vi "Process BMP JPG PNG.vi"() -> ()   [LabVIEW 2015]
uses:
  Typedefs/typedef_enum_ColorSpace.ctl
  Typedefs/typedef_enum_RGB HSL.ctl
panel:
  in  "Threshhold":i32=100
  out "Image_Object":i16[][](graph)
  out "Object(s) Start/Stop/Sum":i32[][](array[numeric])
  in  "cumulative?":bool
  out "RGB/HSL":T1[](array[typedef])=[enum."Red/Hue", enum."Grn/Sat", enum."Blu/Lit"]
  out "Col_Sum":cluster{i32[], "Col_Sum":i16[]}(graph)
  out "Row_Sum":cluster{"Row_Sum":i16[], i32[]}[](graph)
  out "Image_ColorMask":i16[][](graph)
  in  "ColorMask High/Low":u8[][](array[numeric])=[[90, 80], [255, 230], [255, 100]]
  out "Image_Blu/Lit":u8[][](graph)
  out "Image_Grn/Sat":u8[][](graph)
  out "Image_Red/Hue":u8[][](graph)
  out "Picture":picture
  in  "ColorSpace":T2=enum."HSL"
  in  "File Path":path
  # "(.bmp .jpg or .png file)"
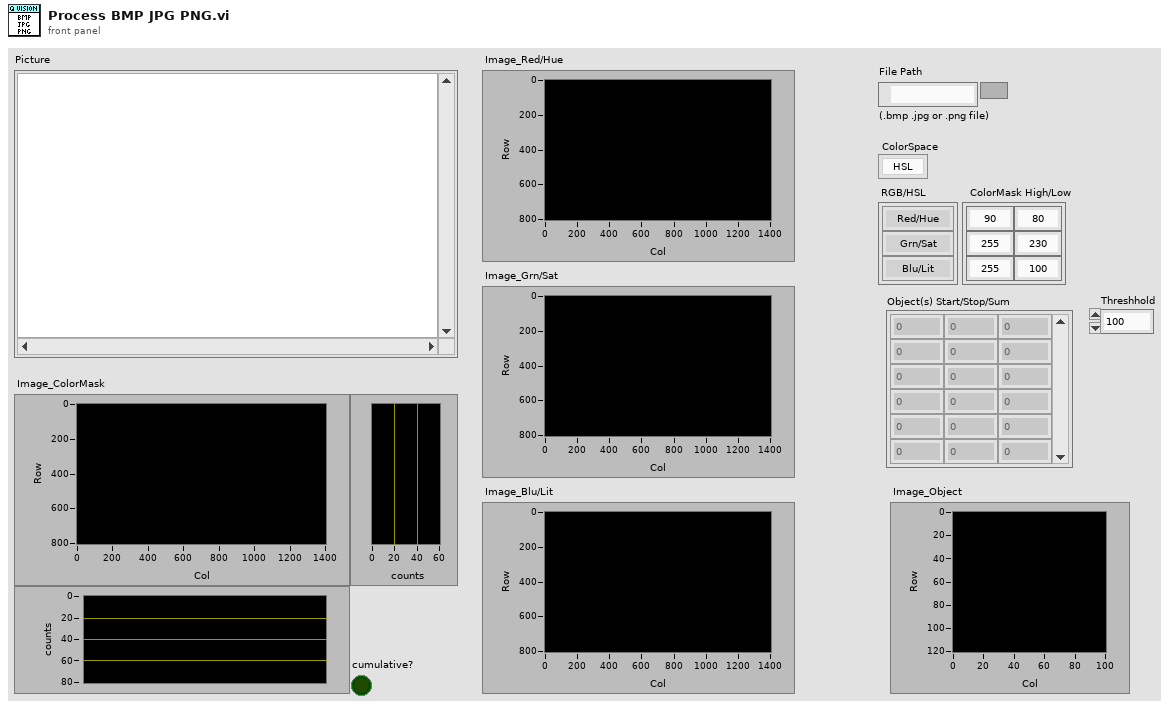
[diagram p1: front panel]
types:
  T1 = typedef "typedef_enum_RGB HSL.ctl" = enum16{"Red/Hue", "Grn/Sat", "Blu/Lit"}
  T2 = typedef "typedef_enum_ColorSpace.ctl" = enum16{"RGB", "HSL"}
  T3 = typedef "imagedata.ctl" = cluster{"image type":i32, "image depth":i32, "image":u8[], "mask":u8[], "colors":u32[], "Rectangle":cluster{"left":i16, "top":i16, "right":i16, "bottom":i16}}
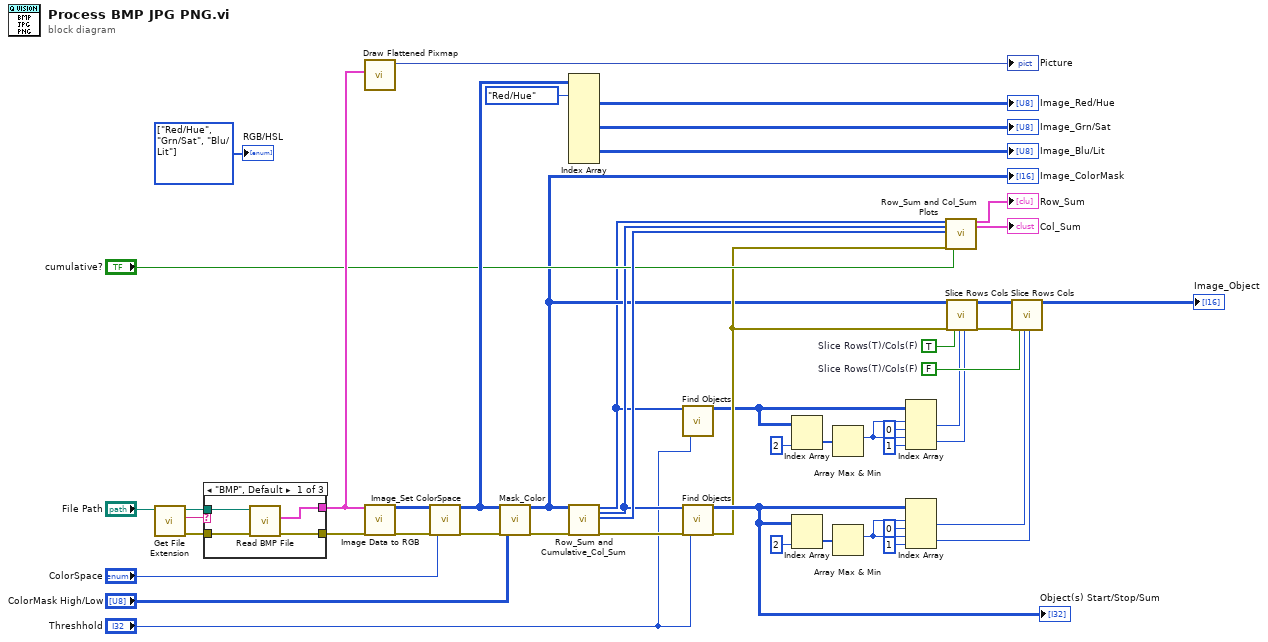
[diagram p0: block diagram]
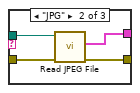
[diagram p2: hidden frame]
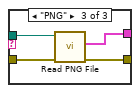
[diagram p3: hidden frame]
diagram:
  w5 = FALSE  # Slice Rows(T)/Cols(F)
  w18 = TRUE  # Slice Rows(T)/Cols(F)
  w31 = T1[] [enum."Red/Hue", enum."Grn/Sat", enum."Blu/Lit"] items=["Red/Hue", "Grn/Sat", "Blu/Lit"]
  n1 = call <vilib>:"Get File Extension.vi"("file"="File Path") -> ("error out"=w47:errorcluster, "lowercase file extension"=w49:string, "dup file"=w48:path)  [unwired: 6 in, 2 out]
  n2 = case shown="\"BMP\", Default" w49 {
    tunnel: w48 -> [w54 w58 w62]
    tunnel: w47 -> [w53 w57 w61]
    tunnel: [w52 w56 w60] -> w43
    tunnel: [w51 w55 w59] -> w46
    frame "BMP", Default {
      n3 = call <vilib>:"Read BMP File.vi"("error in (no error)"=w53, "path to BMP file"=w54) -> ("error out"=w51:errorcluster, "image data"=w52:T3)  [unwired: 7 in, 1 out]
    }
    frame "JPG" {
      n4 = call <vilib>:"Read JPEG File.vi"("error in (no error)"=w57, "path to JPEG file"=w58) -> ("error out"=w55:errorcluster, "image data"=w56:T3)  [unwired: 7 in, 1 out]
    }
    frame "PNG" {
      n5 = call <vilib>:"Read PNG File.vi"("error in (no error)"=w61, "path to PNG file"=w62) -> ("error out"=w59:errorcluster, "image data"=w60:T3)  [unwired: 7 in, 1 out]
    }
  }
  n6 = call <vilib>:"Draw Flattened Pixmap.vi"("image data"=w43) -> ("new picture"=→"Picture":picture)  [unwired: 8 in]
  n7 = call "Image Data to RGB.vi"("image data"=w43, "error in (no error)"=w46) -> ("Image_3d_RGB"=w44:u8[][][], "error out"=w45:errorcluster)  [unwired: 16 in]
  n8 = call "Image_Set ColorSpace.vi"("Image_3d"=w44, "error in (no error)"=w45, "ColorSpace"="ColorSpace") -> ("Image_3d_ColorSpace"=w35:u8[][][], "error out"=w36:errorcluster)  [unwired: 15 in]
  n9 = call "Mask_Color.vi"("Image_3d"=w35, "error in (no error)"=w36, "ColorMask High/Low"="ColorMask High/Low") -> ("Image_2d"=w17:i16[][], "error out"=w32:errorcluster)  [unwired: 15 in]
  "Image_ColorMask" <- w17
  n10 = Index Array(array=w35, index (dim 0) #1=typedef_enum_RGB_HSL."Red/Hue" ("RGB")) -> (element #1=→"Image_Red/Hue":u8[][], element #2=→"Image_Grn/Sat":u8[][], element #3=→"Image_Blu/Lit":u8[][])  [unwired: 8 in]
  n11 = call "Row_Sum and Cumulative_Col_Sum.vi"("Image_2d"=w17, "error in (no error)"=w32) -> ("Row_Sum"=w16:i16[], "Col_Sum"=w27:i16[], "Cum_Col_Sum"=w29:i16[], "error out"=w20:errorcluster)  [unwired: 14 in]
  n12 = call "Find Objects.vi"("RowSum or ColSum"=w16, "Threshhold"="Threshhold") -> ("Object(s) Start/Stop/Sum"=w10:i32[][])  [unwired: 16 in, 1 out]
  n13 = call "Find Objects.vi"("RowSum or ColSum"=w27, "error in (no error)"=w20, "Threshhold"="Threshhold") -> ("Object(s) Start/Stop/Sum"=w24:i32[][], "error out"=w19:errorcluster)  [unwired: 15 in]
  "Object(s) Start/Stop/Sum" <- w24
  n14 = Index Array(array=w10, index (col)=2 ("disabled index (col)")) -> (element=w12:i32[])  [unwired: 1 in]
  n15 = Index Array(array=w24, index (col)=2 ("disabled index (col)")) -> (element=w25:i32[])  [unwired: 1 in]
  n16 = Array Max & Min(array=w12) -> (max index (indices)=w13:i32)  [unwired: 3 out]
  n17 = Array Max & Min(array=w25) -> (max index (indices)=w23:i32)  [unwired: 3 out]
  n18 = Index Array(array=w10, index (row) #1=w13, index (col) #1=0 ("disabled index (col)"), index (row) #2=w13, index (col) #2=1 ("disabled index (col)")) -> (element #1=w3:i32, element #2=w4:i32)
  n19 = Index Array(array=w24, index (row) #1=w23, index (col) #1=0 ("disabled index (col)"), index (row) #2=w23, index (col) #2=1 ("disabled index (col)")) -> (element #1=w7:i32, element #2=w6:i32)
  n20 = call "Row_Sum and Col_Sum Plots.vi"("Row_Sum"=w16, "Col_Sum"=w27, "Cum_Col_Sum"=w29, "error in (no error)"=w19, "cumulative?"="cumulative?") -> ("Row_Sum Plot"=→"Row_Sum":cluster{"X":i16[], "Y":i32[]}[], "Col_Sum Plot"=→"Col_Sum":cluster{"X":i32[], "Y":i16[]})  [unwired: 12 in, 1 out]
  n21 = call "Slice Rows Cols.vi"("Image_2d"=w17, "error in (no error)"=w19, "Slice Rows(T)/Cols(F)"=w18, "Start Index"=w3, "Stop Index"=w4) -> ("Image_2d_Slice"=w9:i16[][], "error out"=w8:errorcluster)  [unwired: 13 in]
  n22 = call "Slice Rows Cols.vi"("Image_2d"=w9, "error in (no error)"=w8, "Slice Rows(T)/Cols(F)"=w5, "Start Index"=w7, "Stop Index"=w6) -> ("Image_2d_Slice"=→"Image_Object":i16[][])  [unwired: 13 in, 1 out]
  "RGB/HSL" <- w31
